vi "TTLout.vi"(6 "synch_signal":refnum<k21>, 10 "Handshake":refnum<k21>="TTL_Handshake1", 11 "FPGA I/O":refnum<k21>="TTL-out1") -> ()   [LabVIEW 2018]
uses:
  <vilib>/Platform/TimedLoop/XDataNode/timing_clust.ctl
  <vilib>/Platform/TimedLoop/XDataNode/nitl_modes.ctl
  <vilib>/Platform/TimedLoop/XDataNode/wakeup.ctl
  <vilib>/rvi/Emulation/niFpgaSctlEmulationGetInTimedLoop.vi
  <vilib>/rvi/Emulation/niFpgaEmulationReportErrorSimple.vi
  <vilib>/rvi/Emulation/niFpgaGetClockAttributes.vi
  <vilib>/rvi/Emulation/niFpgaCriticalErrorInLSC.vi
  <vilib>/rvi/DataTransferAndStorage/Container/Common/niFpgaContainerExecOnDevCompGetState.vi
  <vilib>/rvi/Emulation/niFpgaEmulationIsFPGAContextNoSignature.vi
  <vilib>/rvi/DataTransferAndStorage/Container/Common/niFpgaContainerGetUniqueNameForEmu.vi
  <vilib>/rvi/eio/common/nirviEmuReportErrorAndStop.vi
  <vilib>/rvi/Emulation/niFpgaProcessEmulError.vi
  <vilib>/rvi/eio/common/nirviEmuTemplateMethod_errors.vi
  <vilib>/Platform/TimedLoop/XDataNode/XDataNode.xnode
  <vilib>/rvi/DataTransferAndStorage/Container/XNode/niFpgaContainer.xnode
  <vilib>/rvi/DataTransferAndStorage/Handshake/Emulation/niFpgaHandshakeEmulationRefIn.vi
  <vilib>/eio/EIONode/EIONode.xnode
  <vilib>/Platform/TimedLoop/XDataNode/XDNodeRunTimeDep.lvlib
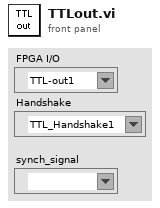
[diagram p1: front panel]
types:
  T1 = typedef "XDNodeRunTimeDep.lvlib/timing_clust.ctl" = cluster{"Expected End [f-1]":u64, "Actual End [f-1]":u64, "Finished Late? [f-1]":bool, "Expected End [i-1]":u64, "Actual End [i-1]":u64, "Finished Late? [i-1]":bool, "Expected Start [i]":u64, "Actual Start [i]":u64, "Expected Start [f]":u64, "Actual Start [f]":u64, "Source Name":string, "Structure Name":string, "Period":i64, "Deadline":i64, "Offset":i64, "Start":i64, "Priority":i32, "Timeout":i32, "Mode":T2, "Wakeup Reason":T3, "Error":errorcluster, "Source Type":string, "Secondary Source Type":string, "Global End Time":u64, "Global Start Time":u64, "Frame Duration":u64, "Iteration Duration":u64, "Assigned CPU":i32, "I/O Scan Engine Mode":u32}
  T2 = typedef "XDNodeRunTimeDep.lvlib/nitl_modes.ctl" = enum32{"No Change", "Process missed periods, maintain original phase", "Discard missed periods, maintain original phase", "Process missed periods, ignore original phase", "Discard missed periods, ignore original phase"}
  T3 = typedef "XDNodeRunTimeDep.lvlib/wakeup.ctl" = enum32{"Normal", "Aborted", "Asynchronous wakeup", "Timing source error", "Timed loop error", "Timeout"}
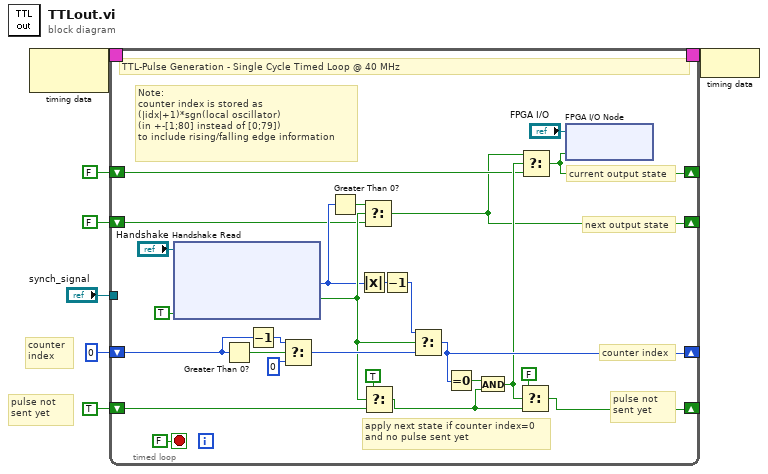
[diagram p0: block diagram]
diagram:
  # "counter \nindex"
  # "pulse not sent yet"
  n1 = node-c288() -> (w7:T1)  [unwired: 1 in]
  n2 = timed-loop {
    timing: w7 -> [_]
    timing-out: [_] -> w6
    shift-right: [w31] -> _
    shift-left: TRUE -> [w30]
    shift-right: [w22] -> _
    shift-left: i8 0 ("Data") -> [w19]
    shift-right: [w18] -> _
    shift-left: FALSE ("t") -> [w11]
    shift-right: [w10] -> _
    shift-left: FALSE ("t") -> [w12]
    tunnel: "synch_signal" -> [_]
    stop <- FALSE stop-if-true
    # "Note: \ncounter index is stored as \n(|idx|+1)*sgn(local oscillator)\n(in +-[1;80] instead of [0;79]) \nto include rising/falling edge information"
    # "apply next state if counter index=0 \nand no pulse sent yet"
    # "current output state"
    # "next output state"
    # "counter index"
    # "pulse not sent yet"
    # "TTL-Pulse Generation - Single Cycle Timed Loop @ 40 MHz"
    n3 = xnode ("Handshake Read")("Ready for Output"=TRUE, "Handshake In"="Handshake") -> ("Data"=w14:i8, "Output Valid"=w15:bool)  [unwired: 1 out]
    n4 = Greater Than 0?(x=w19) -> (x > 0?=w28:bool)
    n5 = Decrement(x=w19) -> (x-1=w27:i8)
    n6 = Select(t=w27, s=w28, f=i8 0) -> (s? t:f=w25:i8)
    n7 = Greater Than 0?(x=w14) -> (x > 0?=w13:bool)
    n8 = Absolute Value(x=w14) -> (abs(x)=w17:i8)
    n9 = Select(t=w13, s=w15, f=w12) -> (s? t:f=w10:bool)
    n10 = Select(t=TRUE, s=w15, f=w30) -> (s? t:f=w24:bool)
    n11 = Decrement(x=w17) -> (x-1=w16:i8)
    n12 = Select(t=w16, s=w15, f=w25) -> (s? t:f=w22:i8)
    n13 = Equal To 0?(x=w22) -> (x = 0?=w23:bool)
    n14 = And(x=w23, y=w24) -> (x .and. y?=w20:bool)
    n15 = Select(t=FALSE, s=w20, f=w24) -> (s? t:f=w31:bool)
    n16 = Select(t=w10, s=w20, f=w11) -> (s? t:f=w18:bool)
    n17 = xnode "FPGA I/O Node"("I/O Item"=w18, "FPGA I/O In"="FPGA I/O") -> ()  [unwired: 1 out]
  }
  n18 = node-c288(w6) -> ()
